vi "Write Picture Control Ref.vi"(8 "error in (no error)":errorcluster, 10 "Picture Control Ref":refnum<vi>, 11 "Reference Control in":refnum<class "Reference Control.lvclass">) -> (0 "error out":errorcluster, 3 "Reference Control out":refnum<class "Reference Control.lvclass">)   [LabVIEW 2016, in "Reference Control.lvclass"]
uses:
  Reference Control.lvclass
  Reference Control.lvclass/Reference Control.ctl
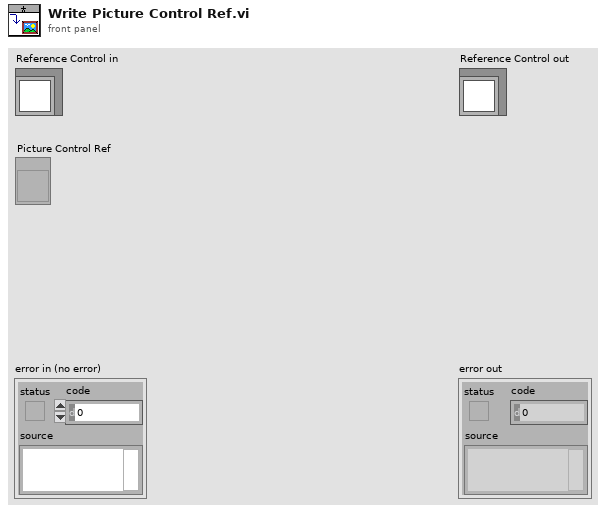
[diagram p1: front panel]
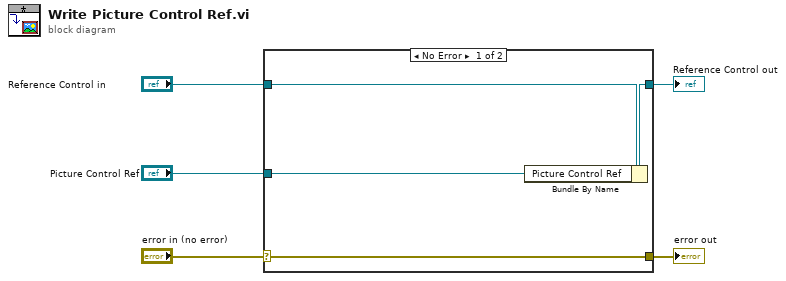
[diagram p0: block diagram]
diagram:
  n1 = case shown="No Error" "error in (no error)" {
    selector: "error in (no error)" -> [w9 w10]
    tunnel: [w9 w10] -> w4
    tunnel: [w7 w11] -> w2
    tunnel: "Reference Control in" -> [w8 w11]
    tunnel: "Picture Control Ref" -> [w6 _]
    frame No Error {
      n2 = Bundle By Name(cluster=w8, "Picture Control Ref"=w6) -> (w7:refnum<class "Reference Control.lvclass">)
    }
    frame Error {
    }
  }
  "error out" <- w4
  "Reference Control out" <- w2
